vi "Tree Control - Traverse Route Group Recursive.vi"(7 "tree refnum":refnum<vi>, 8 "error in (no error)":errorcluster, 10 "parent tag":string, 11 "Route Group":refnum<k7>) -> (0 "error out":errorcluster, 3 "Route Group out":refnum<k7>, 5 "tree refnum out":refnum<vi>)   [LabVIEW 2025, in "Switch Executive Controller UI.lvlib"]
uses:
  Switch Executive Controller UI.lvlib
  <vilib>/SwitchExecutive/niseCfg.llb/niseRouteGroup Get Route Groups.vi
  <vilib>/SwitchExecutive/niseCfg.llb/niseRouteGroup Get Routes.vi
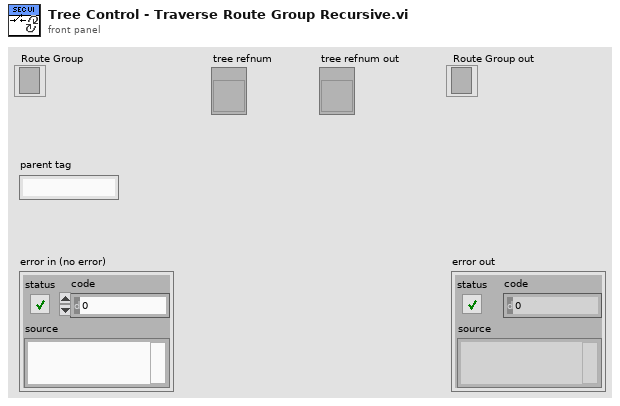
[diagram p1: front panel]
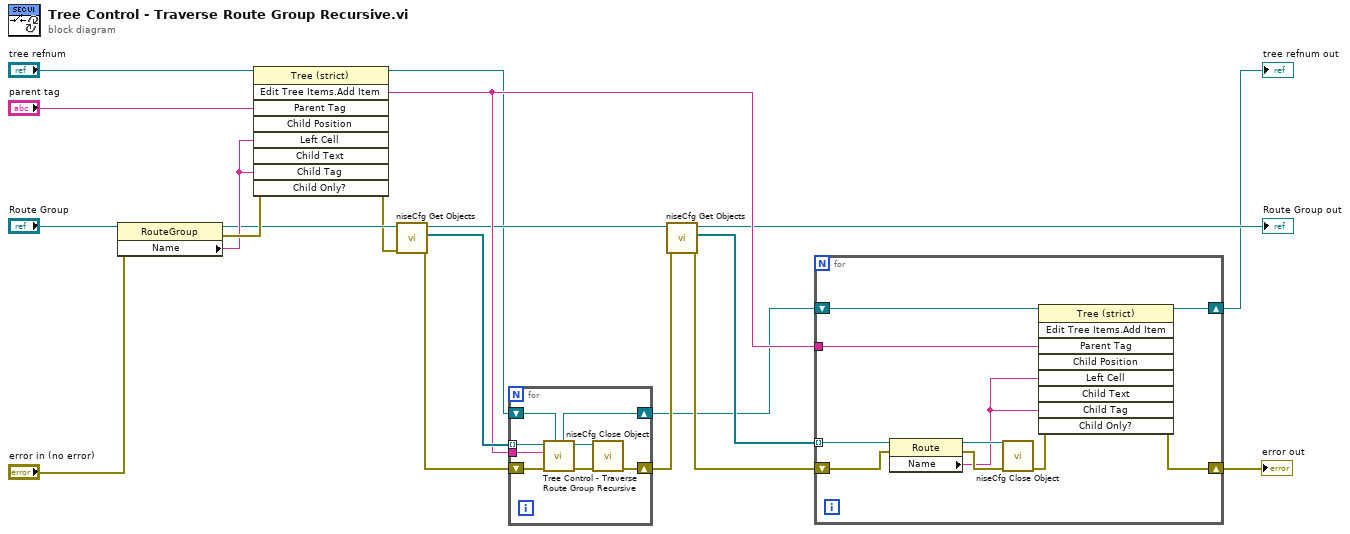
[diagram p0: block diagram]
diagram:
  n1 = property class="RouteGroup"(reference="Route Group", error in="error in (no error)") -> (reference out=w11:refnum<k7>, error out=w14:errorcluster, "Name"=w12:string)
  n2 = invoke class="Tree (strict)" method="Edit Tree Items.Add Item"(reference="tree refnum", error in=w14, "Parent Tag"="parent tag", "Left Cell"=w12, "Child Tag"=w12) -> (reference out=w6:refnum<vi>, error out=w10:errorcluster, "Edit Tree Items:Add Item"=w9:string)  [unwired: 4 in, 6 out]
  n3 = call-poly <vilib>:"niseCfg Get Objects.vi"("error in (no error)"=w10, "Route Group"=w11) -> ("error out"=w15:errorcluster, "Route Groups"=w16:refnum<k7>[], "Route Group out"=w8:refnum<k7>)  [unwired: 7 in]
  n4 = for {
    tunnel: w16 -> [w28] mode=indexing
    shift-right: [w24] -> w7
    shift-left: w15 -> [w27]
    shift-right: [w21] -> w5
    shift-left: w6 -> [w22]
    tunnel: w9 -> [w23]
    n5 = call "Tree Control - Traverse Route Group Recursive.vi"("tree refnum"=w22, "error in (no error)"=w27, "parent tag"=w23, "Route Group"=w28) -> ("error out"=w25:errorcluster, "Route Group out"=w26:refnum<k7>, "tree refnum out"=w21:refnum<vi>)  [unwired: 5 in]
    n6 = call <vilib>:"niseCfg Close Object.vi"("error in (no error)"=w25, "Reference"=w26) -> ("error out"=w24:errorcluster)  [unwired: 9 in]
  }
  n7 = call-poly <vilib>:"niseCfg Get Objects.vi"("error in (no error)"=w7, "Route Group"=w8) -> ("error out"=w19:errorcluster, "Routes"=w20:refnum<k7>[], "Route Group out"=→"Route Group out":refnum<k7>)  [unwired: 7 in]
  n8 = for {
    shift-right: [w31] -> w3
    shift-left: w19 -> [w37]
    tunnel: w20 -> [w38] mode=indexing
    shift-right: [w30] -> w1
    shift-left: w5 -> [w33]
    tunnel: w9 -> [w29]
    n9 = property class="Route"(reference=w38, error in=w37) -> (reference out=w36:refnum<k7>, error out=w35:errorcluster, "Name"=w34:string)
    n10 = call <vilib>:"niseCfg Close Object.vi"("error in (no error)"=w35, "Reference"=w36) -> ("error out"=w32:errorcluster)  [unwired: 9 in]
    n11 = invoke class="Tree (strict)" method="Edit Tree Items.Add Item"(reference=w33, error in=w32, "Parent Tag"=w29, "Left Cell"=w34, "Child Tag"=w34) -> (reference out=w30:refnum<vi>, error out=w31:errorcluster)  [unwired: 4 in, 7 out]
  }
  "error out" <- w3
  "tree refnum out" <- w1
